vi "Main.vi"() -> ()   [LabVIEW 2019]
uses:
  PacDrive.dll
  <instrlib>/Lucam/LVluCam.llb/LuProp.ctl
  <vilib>/MakerHub/LINX/Public/Sensors/Motion/Servo/Servo Set Pulse Width One Channel.vi
  <vilib>/Utility/file.llb/Write Delimited Spreadsheet (string).vi
  Other non home-made vi/PacDrive/PacDrive_x64.dll
  <vilib>/MakerHub/LINX/Public/Utilities/Open Serial.vi
  <vilib>/MakerHub/LINX/Public/Sensors/Motion/Servo/Servo Close One Channel.vi
  <vilib>/MakerHub/LINX/Public/Sensors/Motion/Servo/Servo Open One Channel.vi
  <instrlib>/Lucam/LVluCam.llb/LuFrameFmt.ctl
panel:
  in  "Timer1":bool
  out "Time":string
  out "Path":path
  out "fps 2":dbl
  out "Image":T1(plugin-control)
  in  "Tab Control":T2(tab)
  in  "Box ID 3":enum16{"0", "1", "2"}(ring)=enum."2"
  in  "Valve 16a":bool
  in  "Valve 1a":bool
  in  "Valve 15a":bool
  in  "Valve 14a":bool
  in  "Valve 13a":bool
  in  "Valve 12a":bool
  in  "Valve 11a":bool
  in  "Valve 10a":bool
  in  "Valve 9a":bool
  in  "Valve 7a":bool
  in  "Valve  8a":bool
  in  "Valve 6a":bool
  in  "Valve 5a":bool
  in  "Valve 2a":bool
  in  "Valve 3a":bool
  in  "Valve 4a":bool
  in  "Box ID":enum16{"0", "1", "2"}(ring)
  in  "Valve 16a 2":bool
  in  "Valve 1a 2":bool
  in  "Valve 15a 2":bool
  in  "Valve 14a 2":bool
  in  "Valve 13a 2":bool
  in  "Valve 12a 2":bool
  in  "Valve 11a 2":bool
  in  "Valve 10a 2":bool
  in  "Valve 9a 2":bool
  in  "Valve 7a 2":bool
  in  "Valve  8a 2":bool
  in  "Valve 6a 2":bool
  in  "Valve 5a 2":bool
  in  "Valve 2a 2":bool
  in  "Valve 3a 2":bool
  in  "Valve 4a 2":bool
  in  "Box ID 2":enum16{"0", "1", "2"}(ring)=enum."1"
  in  "stop":bool
  in  "Valve 4a 3":bool
  in  "Valve 3a 3":bool
  in  "Valve 2a 3":bool
  in  "Valve 5a 3":bool
  in  "Valve 6a 3":bool
  in  "Valve  8a 3":bool
  in  "Valve 7a 3":bool
  in  "Valve 9a 3":bool
  in  "Valve 10a 3":bool
  in  "Valve 11a 3":bool
  in  "Valve 12a 3":bool
  in  "Valve 13a 3":bool
  in  "Valve 14a 3":bool
  in  "Valve 15a 3":bool
  in  "Valve 1a 3":bool
  in  "Valve 16a 3":bool
  in  "404":bool
  in  "Record 2":bool
  out "Waiting before toggling":bool
  in  "Wait 3":i32=300
  in  "303":bool
  in  "Automation":bool
  out "ch1-ch2":bool
  in  "Record 1":bool
  in  "ROI 101":cluster{i32, i32, i32, i32}={850, 400, 1300, 600}
  in  "Use threshold 101 i":bool
  in  "Threshold 101 ii":dbl=100.0
  in  "Threshold 101 i":dbl=20.0
  in  "ROI 202a":cluster{i32, i32, i32, i32}={860, 700, 910, 750}
  in  "Threshold 202a":dbl=40.0
  in  "Use threshold 303a i":bool
  in  "Threshold 303a ii":dbl=30.0
  in  "Threshold 303a i":dbl=30.0
  in  "ROI 303a":cluster{i32, i32, i32, i32}={820, 700, 870, 750}
  out "StDev 1":sgl
  out "StDev 1 bar":dbl(slide)=26.100881576538086 scale=20.0..35.0
  out "StDev 202a bar":dbl(slide)=26.100881576538086 scale=20.0..35.0
  out "StDev 202 a":sgl
  out "StDev 303a bar":dbl(slide)=26.100881576538086 scale=20.0..35.0
  out "StDev 303a":sgl
  in  "ROI case":i32
  in  "Threshold multiworm":i32=100
  in  "ROI 303b":cluster{i32, i32, i32, i32}={670, 700, 720, 750}
  in  "Threshold 202b":dbl=40.0
  in  "Threshold 303b":dbl=40.0
  out "StDev 202b bar":dbl(slide)=26.100881576538086 scale=20.0..35.0
  out "StDev 202b":sgl
  out "StDev 303b":sgl
  out "StDev303b bar":dbl(slide)=26.100881576538086 scale=20.0..35.0
  out "Step":string
  in  "Multiworms":bool
  in  "101":bool
  in  "202":bool
  in  "Wait":i32=300
  in  "ROI 202b":cluster{i32, i32, i32, i32}={620, 700, 670, 750}
  out "cmd":bool[](array[boolean])
  in  "Box # & Valve #":T3={[enum."1", enum."1", enum."2", enum."1", enum."1", enum."1", enum."1", enum."2", enum."2", enum."2", enum."1", enum."1", enum."2", enum."2", enum."2", enum."2", enum."2", enum."2", enum."1", enum."1"], [enum."2", enum."3", enum."9", enum."4", enum."1", enum."1", enum."1", enum."1", enum."4", enum."7", enum."7", enum."8", enum."2", enum."3", enum."8", enum."3", enum."5", enum."6", enum."10", enum."7"]}
  in  "Box # => Box IDs":enum16{"0", "1", "2"}[](array[ring])=[enum."0", enum."1", enum."2"]
  out "Valve box ID1":bool[](array[boolean])
  out "Valve box ID0":bool[](array[boolean])
  out "Valve box ID2":bool[](array[boolean])
  in  "Frame Format":T4={"xOffset"=0, "yOffset"=0, "width"=1392, "height"=1040, "pixelFormat"=enum."8 bit", "subSampleX/binningX"=1, "flagsX"=0, "subSampleY/binningY"=1, "flagsY"=0} {"subSampleY/binningY" min=1; "subSampleX/binningX" min=1; "flagsY" items=["none", "Binning"]; "flagsX" items=["none", "Binning"]}
  in  "exposure":sgl=2.0
  in  "fps":i32=10
  in  "gain":sgl
  in  "Serial Port":refnum<visa-resource-name>="COM4"
  in  "Servo Channel":u8=4
  in  "Toggle Reservoir":bool
  in  "Waiting time before toggling reservoir":u32=5000
  in  "Pulse Width (uS)":u16=1100
  in  "Pulse Width (uS) 2":u16=1900
  in  "Initialize Excel file":bool=TRUE
  out "Next step":i32
  out "Init":bool=TRUE
  in  "Step init":i32
  out "Max ROI 101":sgl
  out "Data array 2":string[][](array[string])=[["0", "0"]]
  out "Data array":string[][](array[string])=[["0", "0"]]
  in  "Ch 2":cluster{i32, i32, i32, i32}={50, 650, 450, 1024}
  in  "Ch 1":cluster{i32, i32, i32, i32}={850, 400, 1300, 600}
  out "Save Max ROI 1":bool=TRUE
  out "One shot":bool=TRUE
  out "Movie #":i32
  in  "Close movie 1":bool
  out "New movie 1":bool
  out "Movie Pathway":path=path "C:/Users/Main User/Desktop/Research/Cocktail maker/Experiments/Automation/TEST"
  out "New movie 2":bool
  in  "Close movie 2":bool
  in  "Next1":bool
  # "Box #1 -> ID"
  # "Pressure boxes outputs"
  # "Box #2 -> ID"
  # "Box #3 -> ID"
  # "Oil 1\n\tOil 2\n Oil 3\n Oil 4\n Worm\n\tChemical 1 -buffer\n Chemical 2 \n Valve Oil 1\n Valve Oil 2\n Valve Oil 3\n\tValve Oil 4 Chb1\n Valve Oil 4 Chb2\n Valve worm\n Valve chem 1 - buf\n Valve chem 2\n Valve Outlet 1\n Valve Outlet 2\n Valve Outlet 3\n Valve Outlet 4\n Valve Outlet 5"
  # "Servo motor controls"
  # "Camera parameters"
  # "Automation"
  # "Saving"
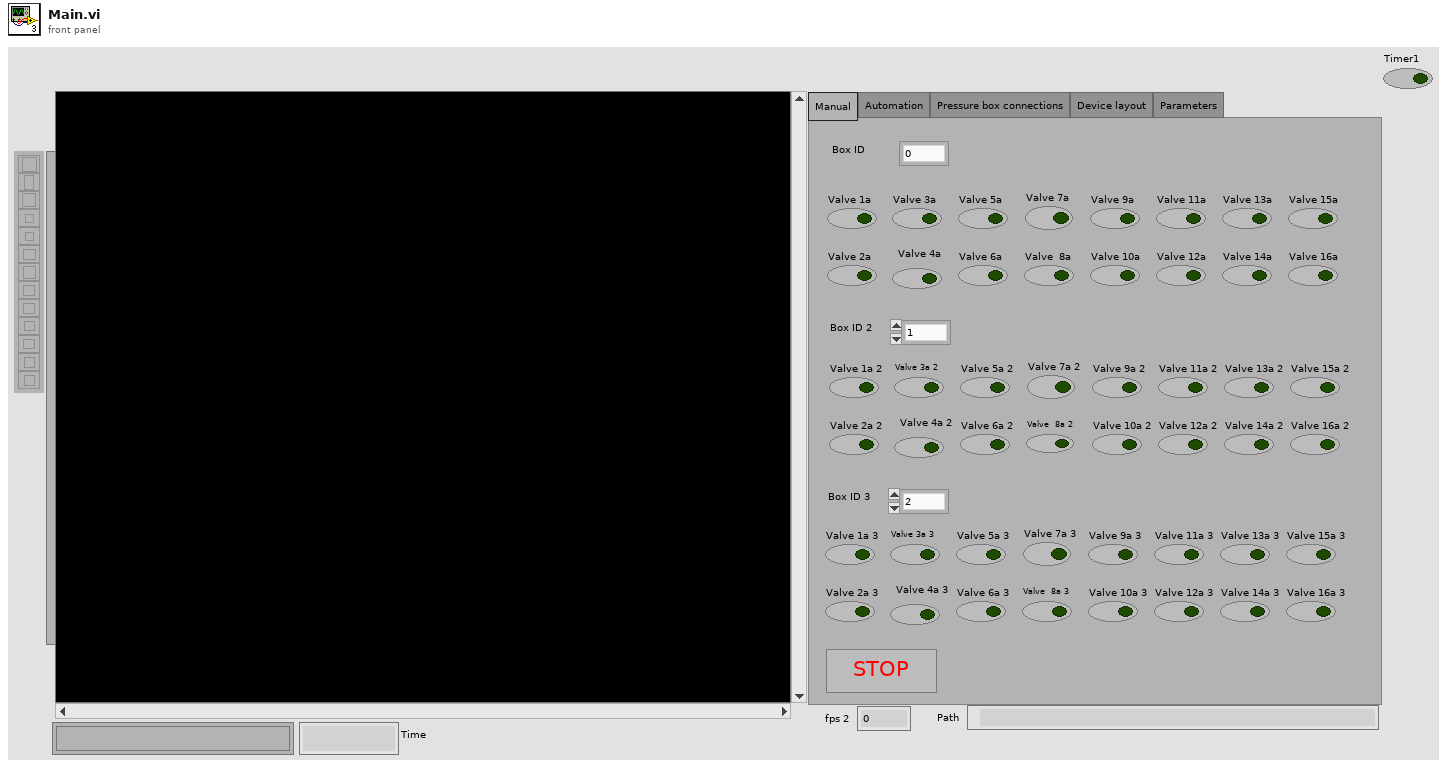
[diagram p1: front panel]
types:
  T1 = typedef "IMAQ Image.ctl" = refnum<image>
  T2 = enum32{"Manual", "Automation", "Pressure box connections", "Device layout", "Parameters"}
  T3 = cluster{enum16{"1", "2", "3"}[], enum16{"1", "2", "3", "4", "5", "6", "7", "8", "9", "10", "11", "12", "13", "14", "15", "16"}[]}
  T4 = typedef "LuFrameFmt.ctl" = cluster{"xOffset":u32, "yOffset":u32, "width":u32, "height":u32, "pixelFormat":enum32{"8 bit", "16 bit", "24 bit RGB", "YUV 422", "Count", "Filter", "32 Bit RGB", "48 Bit RGB"}, "subSampleX/binningX":u16, "flagsX":u16, "subSampleY/binningY":u16, "flagsY":u16}
  T5 = typedef "Image Type" = u32
  T6 = typedef "LuProp.ctl" = u32
  T7 = typedef "LuCamRefnum.ctl" = refnum<k1>
  T8 = cluster{"Fragmentation commands for pressure":cluster{"subarray 2":dbl[][]}[], "Fragmentation commands for waiting times":cluster{"subarray 2":dbl[]}[], "Step list":string[]}
  T9 = cluster{"Fragmentation commands for pressure":cluster{"subarray 2":dbl[][]}[], "Fragmentation commands for waiting times":cluster{"subarray 2":dbl[]}[]}
  T10 = cluster{"New Image":T1, "error out":errorcluster}
  T11 = typedef "IMAQ AVI2 Refnum.ctl" = refnum<k20>
  T12 = typedef "LMH-LINX.lvlib/LINX Ref.ctl" = cluster{"IO":T13, "Interface":T14, "LINX Device Config":T15}
  T13 = typedef "LMH-LINX.lvlib/Platform.ctl" = enum16{"Remote", "Local"}
  T14 = typedef "LMH-LINX.lvlib/Interface.ctl" = enum16{"Serial", "TCP"}
  T15 = typedef "LMH-LINX.lvlib/Device.lvlib/LINX Device Config.ctl" = cluster{"Interface":T14, "COM Port":refnum<visa-resource-name>, "TCP Configuration":T16, "Device Family":u8, "Device ID":u8, "Device Name":string, "TCP Ref":refnum<k5>, "Channels":T17}
  T16 = typedef "LMH-LINX.lvlib/Device.lvlib/TCP Config.ctl" = cluster{"IP Address":string, "Port":u16}
  T17 = typedef "LMH-LINX.lvlib/Channels.ctl" = cluster{"DI":u8[], "DO":u8[], "AI":u8[], "AO":u8[], "PWM":u8[], "QE":u8[], "UART":u8[], "I2C 2":u8[], "SPI":u8[], "CAN":u8[], "Servo":u8[], "AI Ref (V)":dbl, "AI Resolution (Bits)":u8, "AO Ref (V)":dbl, "AO Resolution (Bits)":u8}
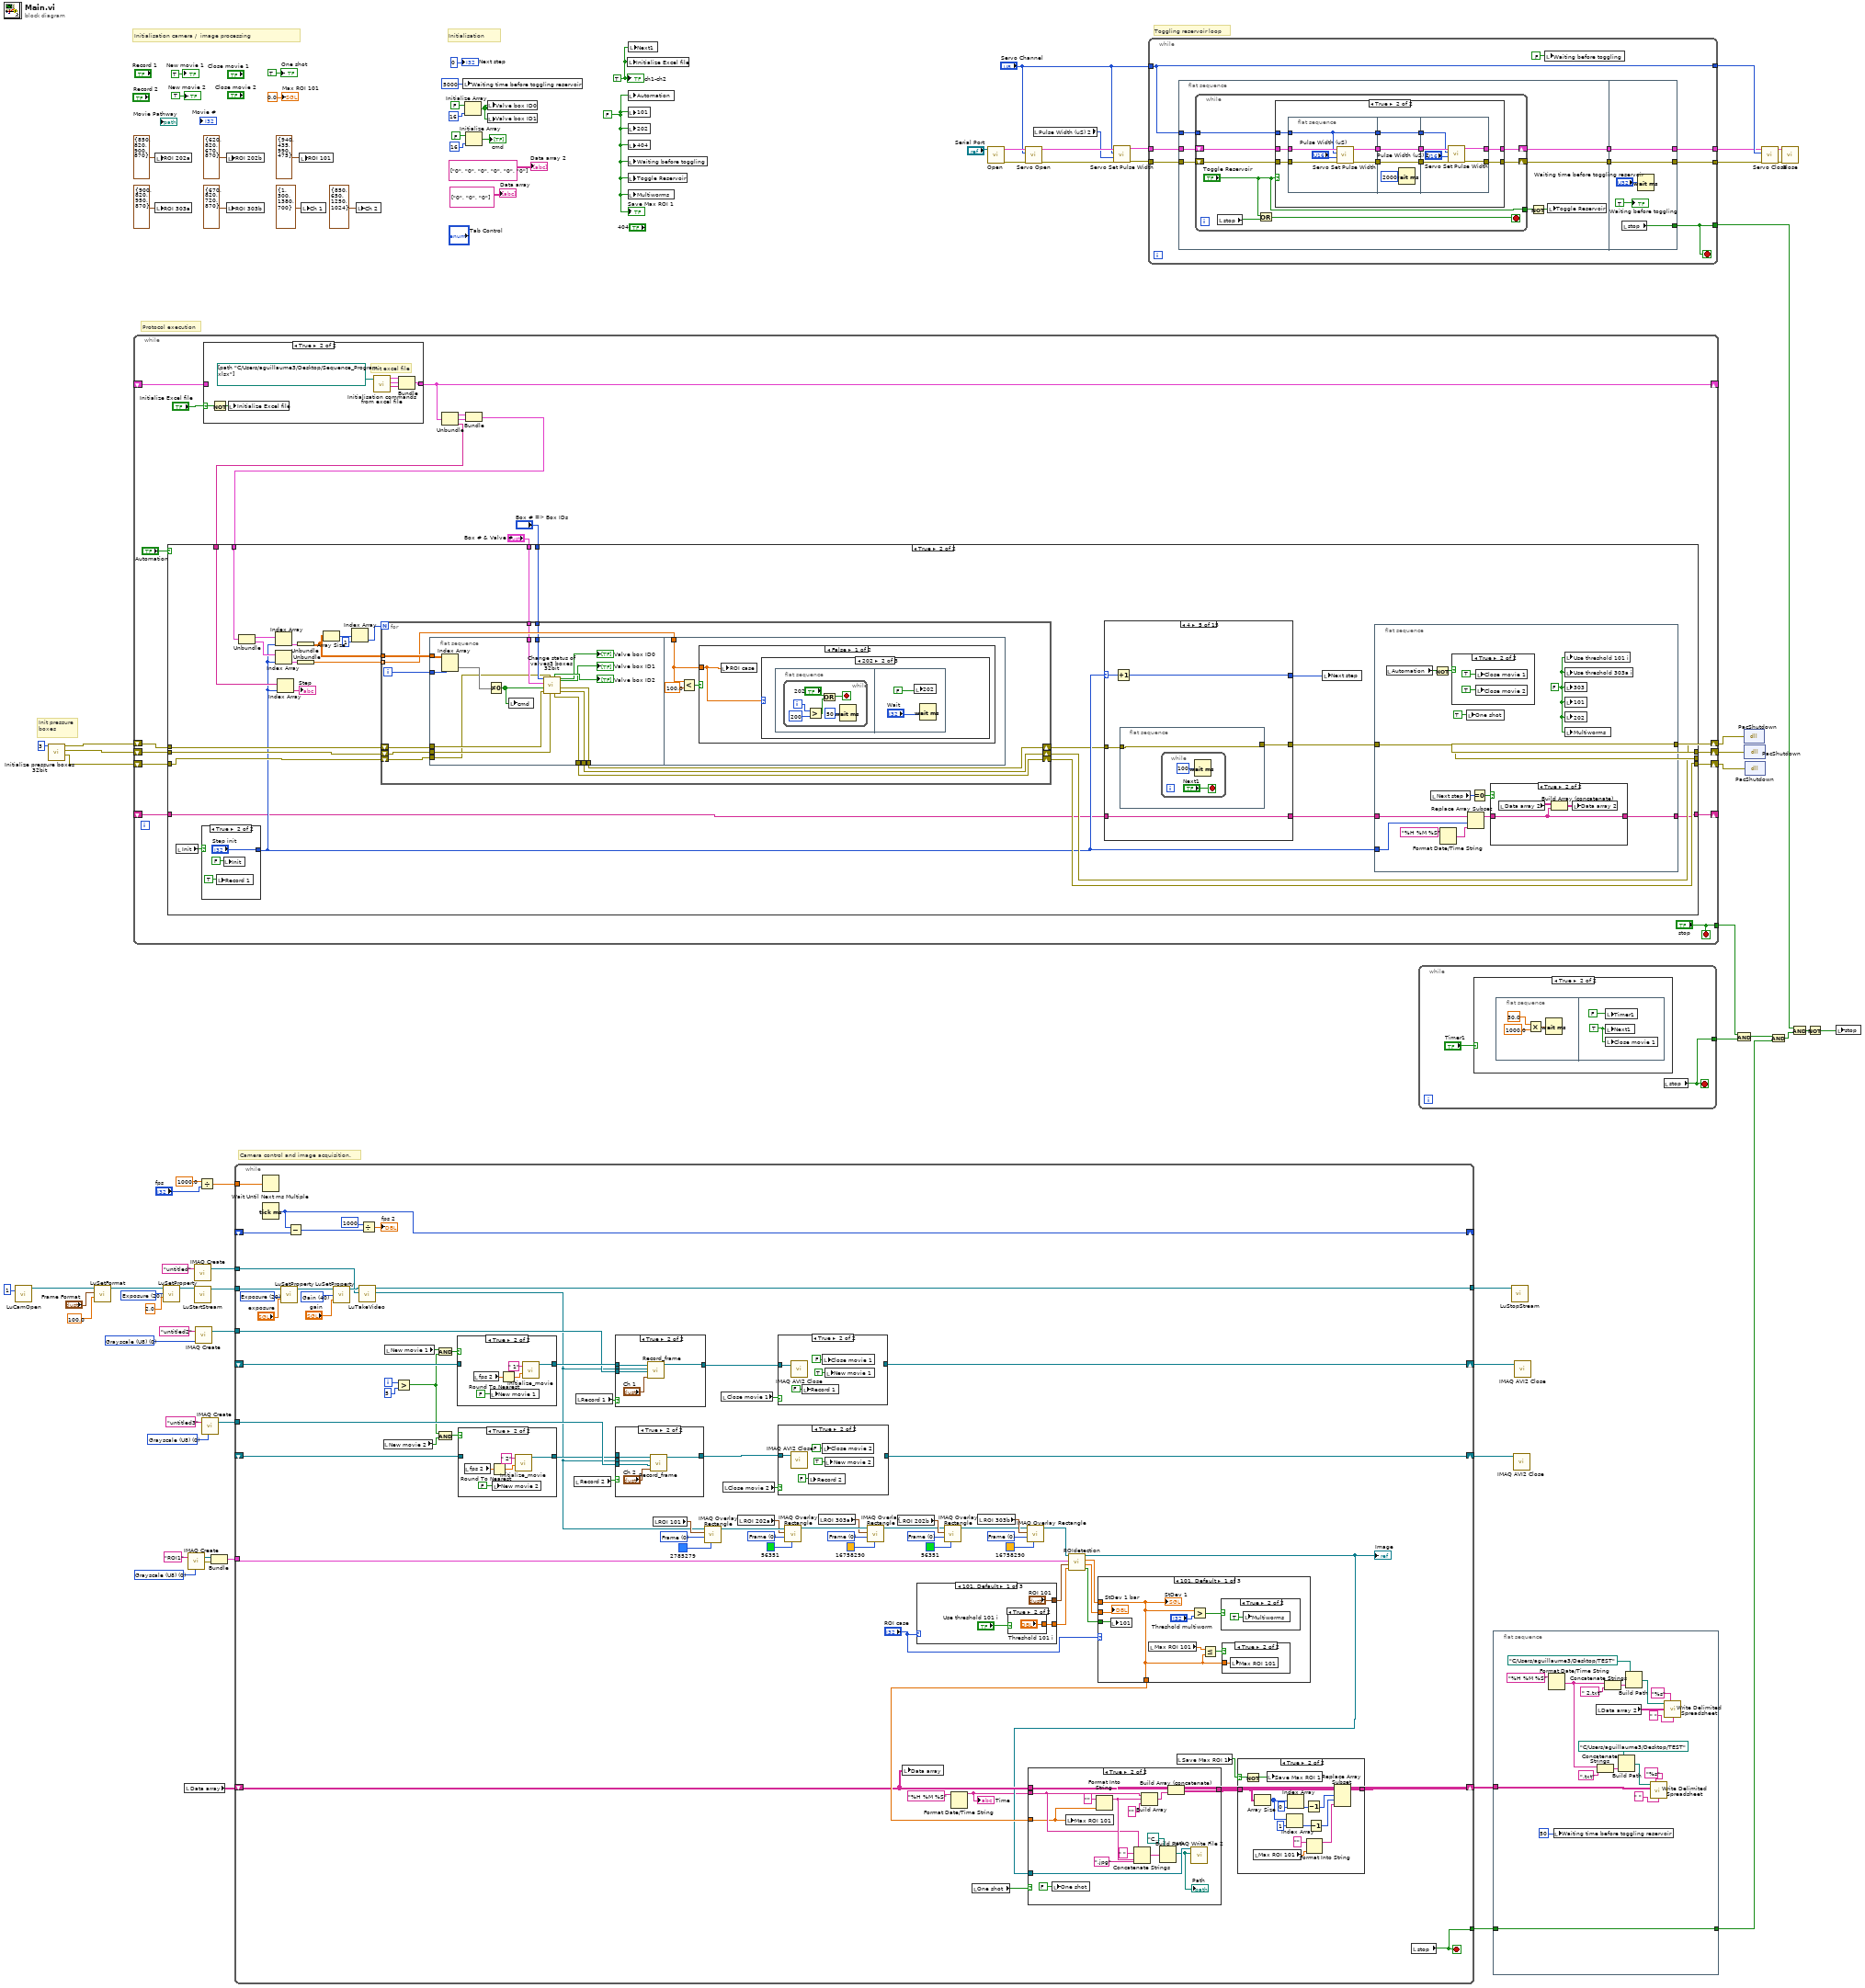
[diagram p0: block diagram]
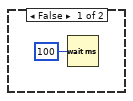
[diagram p2: hidden frame]
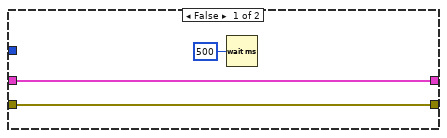
[diagram p3: hidden frame]
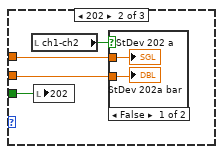
[diagram p13: hidden frame]
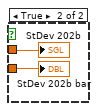
[diagram p14: hidden frame]
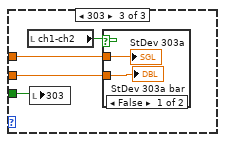
[diagram p15: hidden frame]
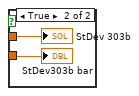
[diagram p16: hidden frame]
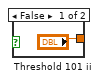
[diagram p17: hidden frame]
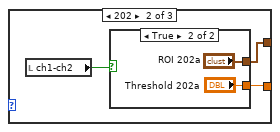
[diagram p18: hidden frame]
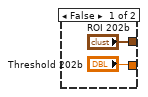
[diagram p19: hidden frame]
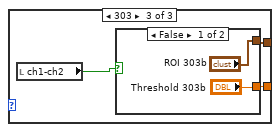
[diagram p20: hidden frame]
diagram:
  w5 = FALSE ("ch1-ch2")
  w25 = T5 0 items=["Grayscale (U8)", "Grayscale (I16)", "Grayscale (SGL)", "Complex (CSG)", "RGB (U32)", "HSL (U32)", "RGB (U64)", "Grayscale (U16)"] ("Image Type")
  w26 = T5 0 items=["Grayscale (U8)", "Grayscale (I16)", "Grayscale (SGL)", "Complex (CSG)", "RGB (U32)", "HSL (U32)", "RGB (U64)", "Grayscale (U16)"] ("Image Type")
  w27 = T5 0 items=["Grayscale (U8)", "Grayscale (I16)", "Grayscale (SGL)", "Complex (CSG)", "RGB (U32)", "HSL (U32)", "RGB (U64)", "Grayscale (U16)"] ("Image Type")
  w66 = T6 20 items=["Brightness"=0, "Contrast"=1, "Hue"=2, "Saturation"=3, "Sharpness"=4, "Gamma"=5, "Pan"=16, "Tilt"=17, "Roll"=18, "Zoom"=19, "Exposure"=20, "Iris"=21, "Focus"=22, "Gain"=40, "Gain Red/Magenta"=41, "Gain Blue/Cyan"=42, "Gain Green1/Yellow1"=43, "Gain Green2/Yellow2"=44, "Demosaicing Method"=64, "Correction Matrix"=65, "Flipping"=66, "Digital Whitebalance U"=69, "Digital Whitebalance V"=70, "Digital Gain"=71, "Digital Gain Red"=72, "Digital Gain Green"=73, "Digital Gain Blue"=74, "Color Format"=80, "Max Width"=81, "Max Height"=82, "ABS Focus"=85, "Still Knee1 Exposure"=96, "Still Knee2 Exposure"=97, "Still Knee3 Exposure"=98, "Video Knee"=99, "Threshold"=101, "Auto Exp Target"=103, "Timestamps"=105, "Snapshot Clock Speed"=106, "Auto Exp Maximum"=107, "Temperature"=108, "Trigger"=110, "Frame Gate"=112, "Exposure Interval"=113, "PWM"=114, "Memory"=115, "Still Strobe Duration"=116, "Fan"=118, "Sync Mode"=119, "Snapshot Count"=120, "LSC X"=121, "LSC Y"=122] ("Property")
  w4 = TRUE ("ch1-ch2")
  # "Camera control and image acquisition."
  # "Protocol execution"
  # "Initialisation"
  # "Toggling reservoir loop"
  # "Init pressure\nboxes"
  # "Initialisation camera /  image processing"
  n1 = call <instrlib>:"LuCamOpen.vi"("Camera Number"=u32 1) -> ("LuCam Session Out"=w71:T7)  [unwired: 9 in, 1 out]
  n2 = call "Initialize pressure boxes 32bit.vi"("Number of \nPressure Boxes"=3 ("Number of \nPressure Boxes")) -> ("error out Box ID2"=w72:errorcluster, "error out Box ID1"=w74:errorcluster, "error out Box ID0"=w75:errorcluster)  [unwired: 8 in]
  n3 = call <instrlib>:"LuSetFormat.vi"("frameRate"=sgl 100.0, "Frame Format"="Frame Format", "LuCam Session In"=w71) -> ("LuCam Session Out"=w67:T7)  [unwired: 7 in, 1 out]
  n4 = while {
    tunnel: ["stop"] -> w3
    shift-right: [w98] -> w8
    shift-left: w75 -> [w97]
    shift-right: [w96] -> w7
    shift-left: w74 -> [w95]
    shift-right: [w94] -> w6
    shift-left: w72 -> [w93]
    shift-right: [w92] -> _
    shift-left: _ -> [w91]
    shift-right: [w88] -> _
    shift-left: _ -> [w90]
    stop <- "stop" stop-if-true
    n5 = case shown="True" "Initialize Excel file" {
      selector: "Initialize Excel file" -> [_ w108]
      tunnel: [w103 w110] -> w88
      tunnel: w90 -> [w103 _]
      frame False {
      }
      frame True {
        # "Init excel file"
        n6 = Not(x=w108) -> (.not. x?=w109:bool)
        n7 = local write "Initialize Excel file"(w109) -> ()
        n8 = call "Initialisation commands from excel file.vi"("Filepath Program code"=path[] [path "C:/Users/aguillaume3/Desktop/Sequence_Program.xlsx"] ("Filepath")) -> ("Step list"=w104:string[], "Fragmentation commands for waiting times"=w105:cluster{"subarray 2":dbl[]}[], "Fragmentation commands for pressure"=w106:cluster{"subarray 2":dbl[][]}[])  [unwired: 8 in]
        n9 = Bundle("Fragmentation commands for pressure"=w106, "Fragmentation commands for waiting times"=w105, "Step list"=w104) -> (w110:T8)  [unwired: 1 in]
      }
    }
    n10 = Unbundle(w88) -> ("Fragmentation commands for pressure"=w87:cluster{"subarray 2":dbl[][]}[], "Fragmentation commands for waiting times"=w86:cluster{"subarray 2":dbl[]}[], "Step list"=w84:string[])
    n11 = Bundle("Fragmentation commands for pressure"=w87, "Fragmentation commands for waiting times"=w86) -> (w85:T9)  [unwired: 1 in]
    n12 = case shown="True" "Automation" {
      tunnel: w84 -> [_ w221]
      tunnel: w85 -> [_ w207]
      tunnel: "Box # & Valve #" -> [_ w220]
      tunnel: w97 -> [w145 w219]
      tunnel: w95 -> [w146 w218]
      tunnel: "Box # => Box IDs" -> [_ w217]
      tunnel: [w143 w216] -> w98
      tunnel: [w142 w212] -> w96
      tunnel: [w140 w213] -> w94
      tunnel: w93 -> [w139 w214]
      tunnel: [w111 w211] -> w92
      tunnel: w91 -> [w111 w197]
      frame False {
        n13 = Initialize Array("Valve 1a", 1 ("dimension size")) -> (w182:bool[])
        n14 = Insert Into Array(array=w182, new element #1="Valve 2a", new element #2="Valve 3a", new element #3="Valve 4a", new element #4="Valve 5a", new element #5="Valve 6a", new element #6="Valve 7a", new element #7="Valve  8a", new element #8="Valve 9a", new element #9="Valve 10a", new element #10="Valve 11a", new element #11="Valve 12a", new element #12="Valve 13a", new element #13="Valve 14a", new element #14="Valve 15a", new element #15="Valve 16a") -> (w144:bool[])  [unwired: 1 in]
        n15 = Boolean Array To Number(Boolean array=w144) -> (number=w166:u32)
        n16 = To Unsigned Word Integer(number=w166) -> (unsigned 16bit integer=w117:u16)
        n17 = Initialize Array("Valve 1a 2", 1 ("dimension size")) -> (w163:bool[])
        n18 = Insert Into Array(array=w163, new element #1="Valve 2a 2", new element #2="Valve 3a 2", new element #3="Valve 4a 2", new element #4="Valve 5a 2", new element #5="Valve 6a 2", new element #6="Valve 7a 2", new element #7="Valve  8a 2", new element #8="Valve 9a 2", new element #9="Valve 10a 2", new element #10="Valve 11a 2", new element #11="Valve 12a 2", new element #12="Valve 13a 2", new element #13="Valve 14a 2", new element #14="Valve 15a 2", new element #15="Valve 16a 2") -> (w119:bool[])  [unwired: 1 in]
        n19 = Boolean Array To Number(Boolean array=w119) -> (number=w147:u32)
        n20 = To Unsigned Word Integer(number=w147) -> (unsigned 16bit integer=w115:u16)
        n21 = Initialize Array("Valve 1a 3", 1 ("dimension size")) -> (w122:bool[])
        n22 = Insert Into Array(array=w122, new element #1="Valve 2a 3", new element #2="Valve 3a 3", new element #3="Valve 4a 3", new element #4="Valve 5a 3", new element #5="Valve 6a 3", new element #6="Valve 7a 3", new element #7="Valve  8a 3", new element #8="Valve 9a 3", new element #9="Valve 10a 3", new element #10="Valve 11a 3", new element #11="Valve 12a 3", new element #12="Valve 13a 3", new element #13="Valve 14a 3", new element #14="Valve 15a 3", new element #15="Valve 16a 3") -> (w118:bool[])  [unwired: 1 in]
        n23 = Boolean Array To Number(Boolean array=w118) -> (number=w138:u32)
        n24 = To Unsigned Word Integer(number=w138) -> (unsigned 16bit integer=w113:u16)
        n25 = case shown="\"1\"" "Box ID 3" {
          tunnel: w118 -> [w185 w186 w187]
          frame "0", Default {
            n26 = local write "Valve box ID0"(w185) -> ()
          }
          frame "1" {
            n27 = local write "Valve box ID1"(w186) -> ()
          }
          frame "2" {
            n28 = local write "Valve box ID2"(w187) -> ()
          }
        }
        n29 = case shown="\"0\", Default" "Box ID 2" {
          tunnel: w119 -> [w188 w189 w190]
          frame "0", Default {
            n30 = local write "Valve box ID0"(w188) -> ()
          }
          frame "1" {
            n31 = local write "Valve box ID1"(w189) -> ()
          }
          frame "2" {
            n32 = local write "Valve box ID2"(w190) -> ()
          }
        }
        n33 = case shown="\"1\"" "Box ID" {
          tunnel: w144 -> [w191 w192 w193]
          frame "0", Default {
            n34 = local write "Valve box ID0"(w191) -> ()
          }
          frame "1" {
            n35 = local write "Valve box ID1"(w192) -> ()
          }
          frame "2" {
            n36 = local write "Valve box ID2"(w193) -> ()
          }
        }
        n37 = dll-call lib="C:/Users/aguillaume3/Desktop/PacDrive.dll" fn="PacSetLEDStates"(error in=w145, "PacNum"="Box ID", "LEDStates"=w117) -> (error out=w143:errorcluster)  [unwired: 5 in, 1 out]
        n38 = dll-call lib="C:/Users/aguillaume3/Desktop/PacDrive.dll" fn="PacSetLEDStates"(error in=w146, "PacNum"="Box ID 2", "LEDStates"=w115) -> (error out=w142:errorcluster)  [unwired: 5 in, 1 out]
        n39 = dll-call lib="C:/Users/aguillaume3/Desktop/PacDrive.dll" fn="PacSetLEDStates"(error in=w139, "PacNum"="Box ID 3", "LEDStates"=w113) -> (error out=w140:errorcluster)  [unwired: 5 in, 1 out]
        "Init" <- TRUE
      }
      frame True {
        n40 = local read "Init"() -> (w215:bool)
        n41 = case shown="True" w215 {
          tunnel: [w347 "Step init"] -> w199
          frame False {
            n42 = local read "Next step"() -> (w347:i32)
          }
          frame True {
            n43 = local write "Record 1"(TRUE ("Record 1")) -> ()
            n44 = local write "Init"(FALSE) -> ()
          }
        }
        n45 = Unbundle(w207) -> ("Fragmentation commands for pressure"=w206:cluster{"subarray 2":dbl[][]}[], "Fragmentation commands for waiting times"=w205:cluster{"subarray 2":dbl[]}[])
        n46 = Index Array(array=w206, index=w199) -> (element=w204:cluster{"subarray 2":dbl[][]})
        n47 = Index Array(array=w205, index=w199) -> (element=w203:cluster{"subarray 2":dbl[]})
        n48 = Index Array(array=w221, index=w199) -> (element=→"Step":string)
        n49 = Unbundle(w204) -> ("subarray 2"=w209:dbl[][])
        n50 = Unbundle(w203) -> ("subarray 2"=w208:dbl[])
        n51 = Array Size(array=w209) -> (size(s)=w202:i32[])
        n52 = Index Array(array=w202, index=1) -> (element=w210:i32)
        n53 = for {
          N: w210 -> [_]
          tunnel: w209 -> [w302]
          tunnel: w208 -> [w301] mode=indexing
          tunnel: w220 -> [w299]
          shift-right: [w294] -> w195
          shift-left: w219 -> [w298]
          shift-right: [w293] -> w212
          shift-left: w218 -> [w297]
          tunnel: w217 -> [w296]
          shift-right: [w292] -> w213
          shift-left: w214 -> [w295]
          i -> [w300]
          n54 = flat-sequence {
            tunnel: w302 -> [w317]
            tunnel: w300 -> [w316]
            tunnel: w299 -> [w315]
            tunnel: w298 -> [w314]
            tunnel: [w313] -> w294
            tunnel: [w312] -> w293
            tunnel: w297 -> [w311]
            tunnel: w296 -> [w308]
            tunnel: w295 -> [w307]
            tunnel: [w306] -> w292
            tunnel: w301 -> [w318]
            frame #0 {
              n55 = Index Array(array=w317, index (col)=w316) -> (element=w310:dbl[])  [unwired: 1 in]
              n56 = Not Equal To 0?(x=w310) -> (x != 0?=w309:bool[])
              n57 = local write "cmd"(w309) -> ()
              n58 = call "Change status of valves3 boxes 32bit.vi"("error in Box ID1"=w311, "error in Box ID2"=w307, "error in Box ID0"=w314, "Status of inlets and\non-chip valves"=w309, "Box # & Valve #"=w315, "Box # => Box ID"=w308) -> ("error out Box ID1"=w312:errorcluster, "error out Box ID0"=w313:errorcluster, "Valve box ID1"=→"Valve box ID1":bool[], "Valve box ID0"=→"Valve box ID0":bool[], "error out Box ID2"=w306:errorcluster, "Valve box ID2"=→"Valve box ID2":bool[])
            }
            frame #1 {
              n59 = Less?(x=w318, y=100.0) -> (x < y?=w320:bool)
              n60 = case shown="False" w320 {
                tunnel: w318 -> [w321 w344]
                frame False {
                  n61 = local write "ROI case"(w321) -> ()
                  n62 = case shown="202" w321 {
                    frame 101, Default {
                      n63 = while {
                        i -> [w326]
                        stop <- w324 stop-if-true
                        n64 = Greater?(x=w326, y=200) -> (0:w325:bool)
                        n65 = Or(x="101", y=w325) -> (x .or. y?=w324:bool)
                        n66 = Wait (ms)(milliseconds to wait=u32 50) -> ()  [unwired: 1 out]
                      }
                    }
                    frame 202 {
                      n67 = flat-sequence {
                        frame #0 {
                          n68 = while {
                            i -> [w332]
                            stop <- w330 stop-if-true
                            n69 = Greater?(x=w332, y=200) -> (0:w331:bool)
                            n70 = Or(x="202", y=w331) -> (x .or. y?=w330:bool)
                            n71 = Wait (ms)(milliseconds to wait=u32 50) -> ()  [unwired: 1 out]
                          }
                        }
                        frame #1 {
                          n72 = local write "202"(FALSE ("101")) -> ()
                          n73 = Wait (ms)(milliseconds to wait="Wait") -> ()  [unwired: 1 out]
                        }
                      }
                    }
                    frame 303 {
                      n74 = flat-sequence {
                        frame #0 {
                          n75 = while {
                            i -> [w340]
                            stop <- w338 stop-if-true
                            n76 = Greater?(x=w340, y=200) -> (0:w339:bool)
                            n77 = Or(x="303", y=w339) -> (x .or. y?=w338:bool)
                            n78 = Wait (ms)(milliseconds to wait=u32 50) -> ()  [unwired: 1 out]
                          }
                        }
                        frame #1 {
                          n79 = local write "303"(FALSE ("101")) -> ()
                          n80 = Wait (ms)(milliseconds to wait="Wait 3") -> ()  [unwired: 1 out]
                        }
                      }
                    }
                  }
                }
                frame True {
                  n81 = Multiply(x=w344, y=1000.0) -> (x*y=w346:dbl)
                  n82 = Wait (ms)(milliseconds to wait=w346) -> ()  [unwired: 1 out]
                }
              }
            }
          }
        }
        n83 = case shown="4" w199 {
          selector: w199 -> [w226 w234 w238 w240 w246 w252 w258 w262 w266 w270 w273 w279 _ w286 _]
          tunnel: [w225 w233 w237 w239 w245 w251 w257 w261 w265 w269 w272 w278 0 w285 0] -> w198
          tunnel: w197 -> [_ w231 w235 w241 w247 w253 w255 w259 w263 w267 w274 w280 w283 w287 w290]
          tunnel: [w224 w232 w236 w242 w243 w254 w256 w260 w264 w268 w275 w281 w284 w288 w291] -> w196
          tunnel: w195 -> [w224 w232 w236 w242 w244 w254 w256 w260 w264 w268 w275 w281 w284 w288 w291]
          tunnel: [string[] ["0 0 0", "0 0 0", "0 0 0", "0 0 0", "0 0 0", "0 0 0"] ("Data array 2") w231 w235 w241 w247 w253 w255 w259 w263 w267 w274 w280 w283 w287 w290] -> w194
          frame 0, Default {
            n84 = case shown="True" "Multiworms" {
              tunnel: w226 -> [w229 _]
              tunnel: [w228 13] -> w225
              frame False {
                n85 = Increment(x=w229) -> (x+1=w228:i32)
              }
              frame True {
              }
            }
            n86 = local write "Save Max ROI 1"(TRUE ("One shot")) -> ()
          }
          frame 1 {
            n87 = Increment(x=w234) -> (x+1=w233:i32)
          }
          frame 2 {
            n88 = Increment(x=w238) -> (x+1=w237:i32)
          }
          frame 3 {
            n89 = Increment(x=w240) -> (x+1=w239:i32)
          }
          frame 4 {
            n90 = Increment(x=w246) -> (x+1=w245:i32)
            n91 = flat-sequence {
              tunnel: w244 -> [w248]
              tunnel: [w248] -> w243
              frame #0 {
                n92 = while {
                  stop <- "Next1" stop-if-true
                  n93 = Wait (ms)(milliseconds to wait=u32 100) -> ()  [unwired: 1 out]
                }
              }
            }
          }
          frame 5 {
            n94 = Increment(x=w252) -> (x+1=w251:i32)
          }
          frame 6 {
            n95 = Increment(x=w258) -> (x+1=w257:i32)
          }
          frame 7 {
            n96 = Increment(x=w262) -> (x+1=w261:i32)
          }
          frame 8 {
            n97 = Increment(x=w266) -> (x+1=w265:i32)
          }
          frame 9 {
            n98 = Increment(x=w270) -> (x+1=w269:i32)
          }
          frame 10 {
            n99 = Increment(x=w273) -> (x+1=w272:i32)
            n100 = local write "Record 1"(TRUE ("Close movie 1")) -> ()
          }
          frame 11 {
            n101 = Increment(x=w279) -> (x+1=w278:i32)
            n102 = local write "Timer1"(TRUE ("Next1")) -> ()
            n103 = local write "Next1"(FALSE ("Next1")) -> ()
          }
          frame 12 {
          }
          frame 13 {
            n104 = Increment(x=w286) -> (x+1=w285:i32)
          }
          frame 14 {
          }
        }
        n105 = local write "Next step"(w198) -> ()
        n106 = flat-sequence {
          tunnel: [w363] -> w216
          tunnel: w196 -> [w363]
          tunnel: w199 -> [w359]
          tunnel: w194 -> [w358]
          tunnel: [w355] -> w211
          frame #0 {
            w361 = FALSE ("101")
            n107 = local read "Automation"() -> (w352:bool)
            n108 = local read "Next step"() -> (w353:i32)
            n109 = Not(x=w352) -> (.not. x?=w351:bool)
            n110 = Format Date/Time String(time format string (%c)="%H %M %S") -> (date/time string=w357:string)  [unwired: 2 in]
            n111 = case shown="True" w351 {
              frame False {
              }
              frame True {
                n112 = local write "Close movie 1"(TRUE ("202")) -> ()
                n113 = local write "Close movie 2"(TRUE ("202")) -> ()
              }
            }
            n114 = local write "One shot"(TRUE ("One shot")) -> ()
            n115 = Replace Array Subset(array=w358, new element=w357, index=w359) -> (w356:string[])
            n116 = Equal To 0?(x=w353) -> (x = 0?=w354:bool)
            n117 = case shown="True" w354 {
              tunnel: w356 -> [w366 w368]
              tunnel: [w366 w368] -> w355
              frame False {
              }
              frame True {
                n118 = local read "Data array 2"() -> (w369:string[][])
                n119 = Build Array (concatenate)(w369, w368) -> (w367:string[][])
                n120 = local write "Data array 2"(w367) -> ()
              }
            }
            n121 = local write "Use threshold 101 i"(w361) -> ()
            n122 = local write "Use threshold 303a i"(w361) -> ()
            n123 = local write "303"(w361) -> ()
            n124 = local write "101"(w361) -> ()
            n125 = local write "202"(w361) -> ()
            n126 = local write "Multiworms"(w361) -> ()
          }
        }
      }
    }
  }
  n127 = local write "ROI 202a"(cluster{i32, i32, i32, i32} {850, 820, 900, 870} ("ROI 405")) -> ()
  n128 = local write "ROI 303a"(cluster{i32, i32, i32, i32} {900, 820, 950, 870} ("ROI 405")) -> ()
  n129 = call <instrlib>:"LuSetProperty.vi"("Value"=sgl 2.0, "Property"=w66, "LuCam Session In"=w67) -> ("LuCam Session Out"=w64:T7)  [unwired: 7 in, 1 out]
  n130 = local read "Data array"() -> (w40:string[][])
  n131 = call "IMAQ Create"("Image Name"="ROI1", "Image Type"=w25) -> ("New Image"=w55:T1, "error out"=w54:errorcluster)  [unwired: 3 in]
  n132 = call "IMAQ Create"("Image Name"="untitled") -> ("New Image"=w62:T1)  [unwired: 4 in, 1 out]
  n133 = call <instrlib>:"LuStartStream.vi"("LuCam Session In"=w64) -> ("LuCam Session Out"=w63:T7)  [unwired: 9 in, 1 out]
  n134 = call "IMAQ Create"("Image Name"="untitled2", "Image Type"=w27) -> ("New Image"=w34:T1)  [unwired: 3 in, 1 out]
  n135 = Divide(x=1000.0, y="fps") -> (x/y=w58:dbl)
  n136 = call "IMAQ Create"("Image Name"="untitled3", "Image Type"=w26) -> ("New Image"=w29:T1)  [unwired: 3 in, 1 out]
  n137 = Bundle("New Image"=w55, "error out"=w54) -> (w53:T10)  [unwired: 1 in]
  n138 = local write "ROI 202b"(cluster{i32, i32, i32, i32} {620, 820, 670, 870} ("ROI 406")) -> ()
  n139 = local write "ROI 303b"(cluster{i32, i32, i32, i32} {670, 820, 720, 870} ("ROI 406")) -> ()
  n140 = while "Camera control and image acquisition." {
    tunnel: w63 -> [w429]
    tunnel: w62 -> [w430]
    shift-right: [w443] -> _
    shift-left: _ -> [w442]
    tunnel: w58 -> [w441]
    tunnel: [w431] -> w57
    shift-right: [w416] -> w33
    shift-left: _ -> [w414]
    tunnel: [w427] -> w45
    tunnel: w53 -> [w420]
    shift-right: [w418] -> w37
    shift-left: w40 -> [w417]
    tunnel: w34 -> [w412]
    tunnel: w29 -> [w410]
    shift-right: [w405] -> w28
    shift-left: _ -> [w404]
    i -> [w403]
    stop <- w427 stop-if-true
    w382 = u32 0 items=["Frame", "Fill", "Highlight"] ("Drawing Mode (Frame)")
    w379 = u32 0 items=["Frame", "Fill", "Highlight"] ("Drawing Mode (Frame)")
    w387 = u32 0 items=["Frame", "Fill", "Highlight"] ("Drawing Mode (Frame)")
    w390 = u32 0 items=["Frame", "Fill", "Highlight"] ("Drawing Mode (Frame)")
    w396 = u32 0 items=["Frame", "Fill", "Highlight"] ("Drawing Mode (Frame)")
    w435 = T6 40 items=["Brightness"=0, "Contrast"=1, "Hue"=2, "Saturation"=3, "Sharpness"=4, "Gamma"=5, "Pan"=16, "Tilt"=17, "Roll"=18, "Zoom"=19, "Exposure"=20, "Iris"=21, "Focus"=22, "Gain"=40, "Gain Red/Magenta"=41, "Gain Blue/Cyan"=42, "Gain Green1/Yellow1"=43, "Gain Green2/Yellow2"=44, "Demosaicing Method"=64, "Correction Matrix"=65, "Flipping"=66, "Digital Whitebalance U"=69, "Digital Whitebalance V"=70, "Digital Gain"=71, "Digital Gain Red"=72, "Digital Gain Green"=73, "Digital Gain Blue"=74, "Color Format"=80, "Max Width"=81, "Max Height"=82, "ABS Focus"=85, "Still Knee1 Exposure"=96, "Still Knee2 Exposure"=97, "Still Knee3 Exposure"=98, "Video Knee"=99, "Threshold"=101, "Auto Exp Target"=103, "Timestamps"=105, "Snapshot Clock Speed"=106, "Auto Exp Maximum"=107, "Temperature"=108, "Trigger"=110, "Frame Gate"=112, "Exposure Interval"=113, "PWM"=114, "Memory"=115, "Still Strobe Duration"=116, "Fan"=118, "Sync Mode"=119, "Snapshot Count"=120, "LSC X"=121, "LSC Y"=122] ("Property")
    w433 = T6 20 items=["Brightness"=0, "Contrast"=1, "Hue"=2, "Saturation"=3, "Sharpness"=4, "Gamma"=5, "Pan"=16, "Tilt"=17, "Roll"=18, "Zoom"=19, "Exposure"=20, "Iris"=21, "Focus"=22, "Gain"=40, "Gain Red/Magenta"=41, "Gain Blue/Cyan"=42, "Gain Green1/Yellow1"=43, "Gain Green2/Yellow2"=44, "Demosaicing Method"=64, "Correction Matrix"=65, "Flipping"=66, "Digital Whitebalance U"=69, "Digital Whitebalance V"=70, "Digital Gain"=71, "Digital Gain Red"=72, "Digital Gain Green"=73, "Digital Gain Blue"=74, "Color Format"=80, "Max Width"=81, "Max Height"=82, "ABS Focus"=85, "Still Knee1 Exposure"=96, "Still Knee2 Exposure"=97, "Still Knee3 Exposure"=98, "Video Knee"=99, "Threshold"=101, "Auto Exp Target"=103, "Timestamps"=105, "Snapshot Clock Speed"=106, "Auto Exp Maximum"=107, "Temperature"=108, "Trigger"=110, "Frame Gate"=112, "Exposure Interval"=113, "PWM"=114, "Memory"=115, "Still Strobe Duration"=116, "Fan"=118, "Sync Mode"=119, "Snapshot Count"=120, "LSC X"=121, "LSC Y"=122] ("Property")
    n141 = Wait Until Next ms Multiple(millisecond multiple=w441) -> ()  [unwired: 1 out]
    n142 = Tick Count (ms)() -> (millisecond timer value=w443:u32)
    n143 = call <instrlib>:"LuSetProperty.vi"("Value"="exposure", "Property"=w433, "LuCam Session In"=w429) -> ("LuCam Session Out"=w436:T7)  [unwired: 7 in, 1 out]
    n144 = Subtract(x=w443, y=w442) -> (x-y=w440:u32)
    n145 = call <instrlib>:"LuSetProperty.vi"("Value"="gain", "Property"=w435, "LuCam Session In"=w436) -> ("LuCam Session Out"=w432:T7)  [unwired: 7 in, 1 out]
    n146 = call <instrlib>:"LuTakeVideo.vi"("Image In"=w430, "LuCam Session In"=w432) -> ("Image Out"=w384:T1, "LuCam Session Out"=w431:T7)  [unwired: 7 in, 1 out]
    n147 = Divide(x=u32 1000, y=w440) -> (x/y=→"fps 2":dbl)
    n148 = local read "New movie 2"() -> (w398:bool)
    n149 = local read "New movie 1"() -> (w401:bool)
    n150 = Greater?(x=w403, y=5) -> (0:w397:bool)
    n151 = And(x=w401, y=w397) -> (x .and. y?=w400:bool)
    n152 = And(x=w397, y=w398) -> (x .and. y?=w399:bool)
    n153 = case shown="True" w400 {
      tunnel: [w492 w496] -> w415
      tunnel: w414 -> [w492 _]
      frame False {
      }
      frame True {
        n154 = local read "fps 2"() -> (w493:dbl)
        n155 = local write "New movie 1"(FALSE ("New movie")) -> ()
        n156 = Round To Nearest(number=w493) -> (nearest integer value=w494:dbl)
        n157 = call "Initialize_movie.vi"("Frames Per Second"=w494, "Counter"=" 1" ("Ch#")) -> ("AVI Refnum"=w496:T11)  [unwired: 7 in, 2 out]
      }
    }
    n158 = case shown="True" w399 {
      tunnel: [w486 w490] -> w408
      tunnel: w404 -> [w486 _]
      frame False {
      }
      frame True {
        n159 = local read "fps 2"() -> (w487:dbl)
        n160 = Round To Nearest(number=w487) -> (nearest integer value=w488:dbl)
        n161 = local write "New movie 2"(FALSE ("New movie")) -> ()
        n162 = call "Initialize_movie.vi"("Frames Per Second"=w488, "Counter"=" 2" ("Ch#")) -> ("AVI Refnum"=w490:T11)  [unwired: 7 in, 2 out]
      }
    }
    n163 = local read "Record 2"() -> (w411:bool)
    n164 = local read "Record 1"() -> (w428:bool)
    n165 = case shown="True" w428 {
      tunnel: [w550 w555] -> w409
      tunnel: w415 -> [w550 w554]
      tunnel: w384 -> [_ w551]
      tunnel: w412 -> [_ w552]
      frame False {
      }
      frame True {
        n166 = call "Record_frame.vi"("Ch in"="Ch 1", "Image Dst"=w552, "Image Src"=w551, "AVI Refnum in"=w554) -> ("AVI Refnum out"=w555:T11)  [unwired: 6 in, 1 out]
      }
    }
    n167 = case shown="True" w411 {
      tunnel: [w480 w482] -> w406
      tunnel: w408 -> [w480 w483]
      tunnel: w384 -> [_ w485]
      tunnel: w410 -> [_ w484]
      frame False {
      }
      frame True {
        n168 = call "Record_frame.vi"("Ch in"="Ch 2", "Image Dst"=w484, "Image Src"=w485, "AVI Refnum in"=w483) -> ("AVI Refnum out"=w482:T11)  [unwired: 6 in, 1 out]
      }
    }
    n169 = local read "ROI 101"() -> (w394:cluster{i32, i32, i32, i32})
    n170 = call "IMAQ Overlay Rectangle"("Color"=u32 2785279, "Drawing Mode (Frame)"=w396, "Rectangle"=w394, "Image"=w384) -> ("Image Out"=w392:T1)  [unwired: 6 in, 1 out]
    n171 = local read "Close movie 1"() -> (w413:bool)
    n172 = local read "Close movie 2"() -> (w407:bool)
    n173 = local read "ROI 202a"() -> (w391:cluster{i32, i32, i32, i32})
    n174 = case shown="True" w413 {
      tunnel: w409 -> [w498 w502]
      tunnel: [w498 _] -> w416
      frame False {
      }
      frame True {
        n175 = call "IMAQ AVI2 Close"("AVI Refnum"=w502) -> ()  [unwired: 10 in, 1 out]
        n176 = local write "Record 1"(FALSE ("Record")) -> ()
        n177 = local write "Close movie 1"(FALSE ("Close movie")) -> ()
        n178 = local write "New movie 1"(TRUE ("New movie")) -> ()
      }
    }
    n179 = case shown="True" w407 {
      tunnel: w406 -> [w475 w479]
      tunnel: [w475 _] -> w405
      frame False {
      }
      frame True {
        n180 = call "IMAQ AVI2 Close"("AVI Refnum"=w479) -> ()  [unwired: 10 in, 1 out]
        n181 = local write "Record 2"(FALSE ("Record")) -> ()
        n182 = local write "Close movie 2"(FALSE ("Close movie")) -> ()
        n183 = local write "New movie 2"(TRUE ("New movie")) -> ()
      }
    }
    n184 = call "IMAQ Overlay Rectangle"("Color"=u32 56351, "Drawing Mode (Frame)"=w390, "Rectangle"=w391, "Image"=w392) -> ("Image Out"=w393:T1)  [unwired: 6 in, 1 out]
    n185 = local read "ROI 303a"() -> (w388:cluster{i32, i32, i32, i32})
    n186 = call "IMAQ Overlay Rectangle"("Color"=u32 16758290, "Drawing Mode (Frame)"=w387, "Rectangle"=w388, "Image"=w393) -> ("Image Out"=w376:T1)  [unwired: 6 in, 1 out]
    n187 = local read "ROI 202b"() -> (w378:cluster{i32, i32, i32, i32})
    n188 = local write "Data array"(w417) -> ()
    n189 = case shown="101, Default" "ROI case" {
      tunnel: ["ROI 101" w535 w542] -> w421
      tunnel: [w528 w534 w541] -> w422
      frame 101, Default {
        n190 = case shown="True" "Use threshold 101 i" {
          tunnel: ["Threshold 101 ii" "Threshold 101 i"] -> w528
          frame False {
          }
          frame True {
          }
        }
      }
      frame 202 {
        n191 = local read "ch1-ch2"() -> (w533:bool)
        n192 = case shown="True" w533 {
          tunnel: ["ROI 202b" "ROI 202a"] -> w535
          tunnel: ["Threshold 202b" "Threshold 202a"] -> w534
          frame False {
          }
          frame True {
          }
        }
      }
      frame 303 {
        n193 = local read "ch1-ch2"() -> (w540:bool)
        n194 = case shown="False" w540 {
          tunnel: ["ROI 303b" "ROI 303a"] -> w542
          tunnel: ["Threshold 303b" w546] -> w541
          frame False {
          }
          frame True {
            n195 = case shown="False" "Use threshold 303a i" {
              tunnel: ["Threshold 303a ii" "Threshold 303a i"] -> w546
              frame False {
              }
              frame True {
              }
            }
          }
        }
      }
    }
    n196 = call "IMAQ Overlay Rectangle"("Color"=u32 56351, "Drawing Mode (Frame)"=w379, "Rectangle"=w378, "Image"=w376) -> ("Image Out"=w377:T1)  [unwired: 6 in, 1 out]
    n197 = Format Date/Time String(time format string (%c)="%H %M %S") -> (date/time string=w373:string)  [unwired: 2 in]
    "Time" <- w373
    n198 = local read "One shot"() -> (w370:bool)
    n199 = local read "ROI 303b"() -> (w381:cluster{i32, i32, i32, i32})
    n200 = call "IMAQ Overlay Rectangle"("Color"=u32 16758290, "Drawing Mode (Frame)"=w382, "Rectangle"=w381, "Image"=w377) -> ("Image Out"=w375:T1)  [unwired: 6 in, 1 out]
    n201 = call "ROIdetection.vi"("Threshold"=w422, "ROI rect"=w421, "Img Dst"=w420, "Image In"=w375) -> ("condition"=w425:bool, "StDev bar"=w424:dbl, "StDev num"=w423:sgl, "Image Out"=w385:T1)  [unwired: 4 in]
    "Image" <- w385
    n202 = case shown="101, Default" "ROI case" {
      tunnel: w423 -> [w503 w515 w522]
      tunnel: w424 -> [w509 w514 w521]
      tunnel: w425 -> [w508 w512 w523]
      tunnel: [w503 _ _] -> w419
      frame 101, Default {
        n203 = local write "101"(w508) -> ()
        n204 = local read "Max ROI 101"() -> (w504:sgl)
        n205 = Greater?(x=w503, y="Threshold multiworm") -> (0:w507:bool)
        n206 = Less Or Equal?(x=w504, y=w503) -> (x <= y?=w505:bool)
        n207 = case shown="True" w507 {
          frame False {
          }
          frame True {
            n208 = local write "Multiworms"(TRUE ("Multiworms")) -> ()
          }
        }
        n209 = case shown="True" w505 {
          tunnel: w503 -> [_ w510]
          frame False {
          }
          frame True {
            n210 = local write "Max ROI 101"(w510) -> ()
          }
        }
        "StDev 1 bar" <- w509
        "StDev 1" <- w503
      }
      frame 202 {
        n211 = local read "ch1-ch2"() -> (w513:bool)
        n212 = local write "202"(w512) -> ()
        n213 = case shown="False" w513 {
          tunnel: w515 -> [w517 w519]
          tunnel: w514 -> [w516 w518]
          frame False {
            "StDev 202 a" <- w517
            "StDev 202a bar" <- w516
          }
          frame True {
            "StDev 202b" <- w519
            "StDev 202b bar" <- w518
          }
        }
      }
      frame 303 {
        n214 = local read "ch1-ch2"() -> (w520:bool)
        n215 = local write "303"(w523) -> ()
        n216 = case shown="False" w520 {
          tunnel: w522 -> [w525 w527]
          tunnel: w521 -> [w524 w526]
          frame False {
            "StDev 303a" <- w525
            "StDev 303a bar" <- w524
          }
          frame True {
            "StDev303b bar" <- w526
            "StDev 303b" <- w527
          }
        }
      }
    }
    n217 = case shown="True" w370 {
      tunnel: w419 -> [_ w460]
      tunnel: [w459 w473] -> w371
      tunnel: w385 -> [_ w472]
      tunnel: w417 -> [w459 w470]
      tunnel: w373 -> [_ w461]
      frame False {
      }
      frame True {
        n218 = local write "One shot"(FALSE ("One shot")) -> ()
        n219 = local write "Max ROI 101"(w460) -> ()
        n220 = Format Into String(initial string="", w460) -> (resulting string=w464:string)  [unwired: 2 in, 1 out]
        n221 = Concatenate Strings(w461, " " ("initial string"), w464, ".jpg" ("string")) -> (w468:string)
        n222 = Build Array(w461, w464, "" ("element")) -> (w462:string[])
        n223 = Build Path(base path=path "C:/Users/aguillaume3/Desktop/TEST/Pictures", name or relative path=w468) -> (appended path=w469:path)
        "Path" <- w469
        n224 = Build Array (concatenate)(w470, w462) -> (w473:string[][])
        n225 = call-poly "IMAQ Write File 2"("File Path"=w469, "Image"=w472) -> ()  [unwired: 8 in, 2 out]
      }
    }
    n226 = local read "Save Max ROI 1"() -> (w372:bool)
    n227 = case shown="True" w372 {
      selector: w372 -> [_ w450]
      tunnel: w371 -> [w444 w452]
      tunnel: [w444 w451] -> w418
      frame False {
      }
      frame True {
        n228 = Not(x=w450) -> (.not. x?=w449:bool)
        n229 = local read "Max ROI 101"() -> (w455:sgl)
        n230 = Array Size(array=w452) -> (size(s)=w456:i32[])
        n231 = local write "Save Max ROI 1"(w449) -> ()
        n232 = Index Array(array=w456, index=1) -> (element=w448:i32)
        n233 = Index Array(array=w456, index=0) -> (element=w445:i32)
        n234 = Decrement(x=w445) -> (x-1=w446:i32)
        n235 = Format Into String(initial string="", w455) -> (resulting string=w453:string)  [unwired: 2 in, 1 out]
        n236 = Decrement(x=w448) -> (x-1=w447:i32)
        n237 = Replace Array Subset(array=w452, new element=w453, index (row)=w446, index (col)=w447) -> (w451:string[][])
      }
    }
    n238 = local read "stop"() -> (w427:bool)
  }
  n239 = local write "ROI 101"(cluster{i32, i32, i32, i32} {940, 435, 990, 475} ("ROI 406")) -> ()
  n240 = local write "Ch 1"(cluster{i32, i32, i32, i32} {1, 300, 1380, 700} ("ROI 406")) -> ()
  n241 = local write "Ch 2"(cluster{i32, i32, i32, i32} {850, 650, 1250, 1024} ("ROI 406")) -> ()
  n242 = local write "Waiting time before toggling reservoir"(u32 5000 ("Waiting time before toggling reservoir")) -> ()
  n243 = Initialize Array(FALSE, 16 ("dimension size")) -> (w78:bool[])
  n244 = Initialize Array(FALSE, 16 ("dimension size")) -> (→"cmd":bool[])
  n245 = local write "Valve box ID0"(w78) -> ()
  n246 = local write "Valve box ID1"(w78) -> ()
  n247 = local write "Initialize Excel file"(w4) -> ()
  n248 = local write "Automation"(w5) -> ()
  n249 = local write "101"(w5) -> ()
  n250 = local write "202"(w5) -> ()
  n251 = local write "404"(w5) -> ()
  n252 = local write "Waiting before toggling"(w5) -> ()
  n253 = local write "Toggle Reservoir"(w5) -> ()
  n254 = local write "Multiworms"(w5) -> ()
  n255 = local write "Next1"(w4) -> ()
  n256 = call-poly <vilib>:"Open.vi"("Serial Port"="Serial Port") -> ("Error Out"=w21:errorcluster, "LINX Resource"=w22:T12)  [unwired: 8 in, 1 out]
  n257 = call-poly <vilib>:"Servo Open.vi"("Error In"=w21, "Servo Channel"="Servo Channel", "LINX Resource"=w22) -> ("Error Out"=w13:errorcluster, "LINX Resource"=w14:T12)  [unwired: 7 in]
  n258 = local read "Pulse Width (uS) 2"() -> (w11:u16)
  n259 = call-poly <vilib>:"Servo Set Pulse Width.vi"("Error In"=w13, "Pulse Width (uS)"=w11, "Servo Channel"="Servo Channel", "LINX Resource"=w14) -> ("Error Out"=w15:errorcluster, "LINX Resource"=w16:T12)  [unwired: 6 in]
  n260 = while {
    tunnel: [w564] -> w18
    tunnel: w16 -> [w563]
    tunnel: w15 -> [w562]
    tunnel: [w561] -> w17
    tunnel: "Servo Channel" -> [w560]
    tunnel: [w560] -> w19
    tunnel: [w556] -> w9
    stop <- w556 stop-if-true
    n261 = flat-sequence {
      tunnel: w563 -> [w570]
      tunnel: w562 -> [w569]
      tunnel: w560 -> [w567]
      tunnel: [w571] -> w559
      tunnel: [w568] -> w558
      tunnel: [w613] -> w561
      tunnel: [w614] -> w564
      tunnel: w559 -> [w614]
      tunnel: w558 -> [w613]
      tunnel: [w611] -> w556
      frame #0 {
        n262 = while {
          tunnel: w567 -> [w575]
          shift-right: [w579] -> w571
          shift-left: w570 -> [w578]
          shift-right: [w576] -> w568
          shift-left: w569 -> [w577]
          tunnel: ["Toggle Reservoir"] -> w565
          stop <- w573 stop-if-true
          n263 = local read "stop"() -> (w574:bool)
          n264 = Or(x="Toggle Reservoir", y=w574) -> (x .or. y?=w573:bool)
          n265 = case shown="True" "Toggle Reservoir" {
            tunnel: [w581 w589] -> w579
            tunnel: w578 -> [w581 w588]
            tunnel: w577 -> [w580 w587]
            tunnel: [w580 w586] -> w576
            tunnel: w575 -> [_ w585]
            frame False {
              n266 = Wait (ms)(milliseconds to wait=u32 500) -> ()  [unwired: 1 out]
            }
            frame True {
              n267 = flat-sequence {
                tunnel: w588 -> [w598]
                tunnel: w587 -> [w597]
                tunnel: [w599] -> w593
                tunnel: [w596] -> w592
                tunnel: w585 -> [w594]
                tunnel: [w594] -> w583
                tunnel: w593 -> [w603]
                tunnel: w592 -> [w602]
                tunnel: [w603] -> w591
                tunnel: [w602] -> w590
                tunnel: [w600] -> w584
                tunnel: w583 -> [w600]
                tunnel: [w605] -> w586
                tunnel: [w606] -> w589
                tunnel: w591 -> [w608]
                tunnel: w590 -> [w607]
                tunnel: w584 -> [w604]
                frame #0 {
                  n268 = call-poly <vilib>:"Servo Set Pulse Width.vi"("Error In"=w597, "Pulse Width (uS)"="Pulse Width (uS)", "Servo Channel"=w594, "LINX Resource"=w598) -> ("Error Out"=w596:errorcluster, "LINX Resource"=w599:T12)  [unwired: 6 in]
                }
                frame #1 {
                  n269 = Wait (ms)(milliseconds to wait=u32 2000) -> ()  [unwired: 1 out]
                }
                frame #2 {
                  n270 = call-poly <vilib>:"Servo Set Pulse Width.vi"("Error In"=w607, "Pulse Width (uS)"="Pulse Width (uS) 2", "Servo Channel"=w604, "LINX Resource"=w608) -> ("Error Out"=w605:errorcluster, "LINX Resource"=w606:T12)  [unwired: 6 in]
                }
              }
            }
          }
        }
        n271 = Not(x=w565) -> (.not. x?=w566:bool)
        n272 = local write "Toggle Reservoir"(w566) -> ()
      }
      frame #1 {
        n273 = local read "stop"() -> (w611:bool)
        n274 = Wait (ms)(milliseconds to wait="Waiting time before toggling reservoir") -> ()  [unwired: 1 out]
        "Waiting before toggling" <- TRUE ("Waiting before toggling")
      }
    }
    n275 = local write "Waiting before toggling"(FALSE ("Waiting before toggling")) -> ()
  }
  n276 = while {
    tunnel: [w616] -> w1
    stop <- w616 stop-if-true
    n277 = case shown="True" "Timer1" {
      frame False {
        n278 = Wait (ms)(milliseconds to wait=u32 100) -> ()  [unwired: 1 out]
      }
      frame True {
        n279 = flat-sequence {
          frame #0 {
            n280 = Multiply(x=30.0, y=1000.0) -> (x*y=w620:dbl)
            n281 = Wait (ms)(milliseconds to wait=w620) -> ()  [unwired: 1 out]
          }
          frame #1 {
            w621 = TRUE ("stop")
            n282 = local write "Timer1"(FALSE ("Timer1")) -> ()
            n283 = local write "Next1"(w621) -> ()
            n284 = local write "Close movie 1"(w621) -> ()
          }
        }
      }
    }
    n285 = local read "stop"() -> (w616:bool)
  }
  n286 = flat-sequence {
    tunnel: w45 -> [w640]
    tunnel: [w640] -> w44
    tunnel: w37 -> [w623]
    frame #0 {
      n287 = Format Date/Time String(time format string (%c)="%H %M %S") -> (date/time string=w624:string)  [unwired: 2 in]
      n288 = local write "Waiting time before toggling reservoir"(u32 50 ("Waiting time before toggling reservoir")) -> ()
      n289 = local read "Data array 2"() -> (w638:string[][])
      n290 = Concatenate Strings(w624, ".txt" ("initial string")) -> (w630:string)
      n291 = Concatenate Strings(w624, " 2.txt" ("initial string")) -> (w637:string)
      n292 = Build Path(base path=path "C:/Users/aguillaume3/Desktop/TEST", name or relative path=w630) -> (appended path=w628:path)
      n293 = Build Path(base path=path "C:/Users/aguillaume3/Desktop/TEST", name or relative path=w637) -> (appended path=w635:path)
      n294 = call-poly <vilib>:"Write Delimited Spreadsheet.vi"("file path (dialog if empty)"=w628, "format (%s)"="%s", "2D data"=w623, "delimiter (\\t)"=" " ("delimiter (\\t)")) -> ()  [unwired: 10 in, 2 out]
      n295 = call-poly <vilib>:"Write Delimited Spreadsheet.vi"("file path (dialog if empty)"=w635, "format (%s)"="%s", "2D data"=w638, "delimiter (\\t)"=" " ("delimiter (\\t)")) -> ()  [unwired: 10 in, 2 out]
    }
  }
  n296 = call <instrlib>:"LuStopStream.vi"("LuCam Session In"=w57) -> ()  [unwired: 9 in, 2 out]
  n297 = call "IMAQ AVI2 Close"("AVI Refnum"=w28) -> ()  [unwired: 10 in, 1 out]
  n298 = call "IMAQ AVI2 Close"("AVI Refnum"=w33) -> ()  [unwired: 10 in, 1 out]
  n299 = And(x=w3, y=w1) -> (x .and. y?=w2:bool)
  n300 = dll-call lib="C:/Users/aubry/Desktop/Asterix/Research/1. Writing Nat. Comm. Paper/Data/LabVIEW/For paper/LabVIEW for Chemical Profiles in Combining Chamber/Other non home-made vi/PacDrive/PacDrive_x64.dll" fn="PacShutdown"(error in=w8) -> ()  [unwired: 3 in, 2 out]
  n301 = dll-call lib="C:/Users/aubry/Desktop/Asterix/Research/1. Writing Nat. Comm. Paper/Data/LabVIEW/For paper/LabVIEW for Chemical Profiles in Combining Chamber/Other non home-made vi/PacDrive/PacDrive_x64.dll" fn="PacShutdown"(error in=w7) -> ()  [unwired: 3 in, 2 out]
  n302 = dll-call lib="C:/Users/aubry/Desktop/Asterix/Research/1. Writing Nat. Comm. Paper/Data/LabVIEW/For paper/LabVIEW for Chemical Profiles in Combining Chamber/Other non home-made vi/PacDrive/PacDrive_x64.dll" fn="PacShutdown"(error in=w6) -> ()  [unwired: 3 in, 2 out]
  n303 = call-poly <vilib>:"Servo Close.vi"("Error In"=w17, "Servo Channel"=w19, "LINX Resource"=w18) -> ("Error Out"=w24:errorcluster, "LINX Resource"=w23:T12)  [unwired: 7 in]
  n304 = And(x=w2, y=w44) -> (x .and. y?=w10:bool)
  n305 = call <vilib>:"Close.vi"("Error In"=w24, "LINX Resource"=w23) -> ()  [unwired: 9 in, 1 out]
  n306 = And(x=w9, y=w10) -> (x .and. y?=w47:bool)
  n307 = Not(x=w47) -> (.not. x?=w46:bool)
  n308 = local write "stop"(w46) -> ()
  "Next step" <- 0 ("Next step")
  "ch1-ch2" <- w4
  "New movie 1" <- TRUE ("New movie")
  "One shot" <- TRUE ("One shot")
  "Max ROI 101" <- sgl 0.0 ("Max ROI 101")
  "Data array" <- string[][] [["0", "0", "0"]] ("Data array")
  "Save Max ROI 1" <- w5
  "Data array 2" <- string[][] [["0", "0", "0", "0", "0", "0"]] ("Data array 2")
  "New movie 2" <- TRUE ("New movie 2")
